vi "Program Synth.vi"(8 "error in (no error)":errorcluster, 11 "NHMFL Synthesizer in":refnum<class "NHMFL Synthesizer.lvclass">) -> (0 "error out":errorcluster, 3 "NHMFL Synthesizer out":refnum<class "NHMFL Synthesizer.lvclass">)   [LabVIEW 2015, in "NHMFL Synthesizer.lvclass"]
uses:
  NHMFL Synthesizer.lvclass
  NHMFL Synthesizer.lvclass/NHMFL Synthesizer.ctl
  Read NHMFL Synthesizer Configuration.vi
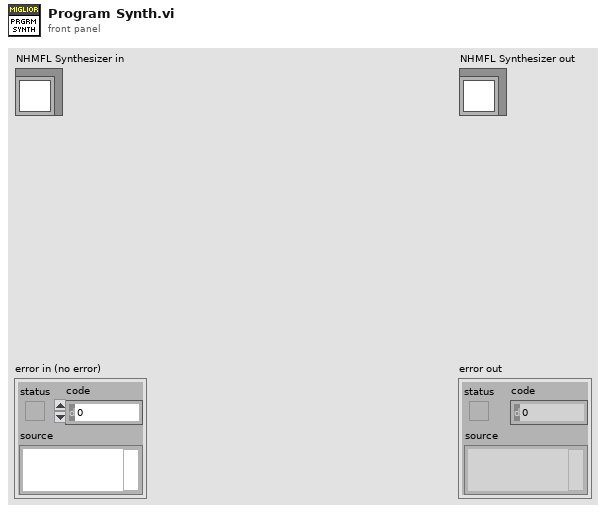
[diagram p1: front panel]
types:
  T1 = typedef "NHMFL Synthesizer Configuration.ctl" = cluster{"DAQmx Device":tag, "Variable amplitude frequency":dbl, "Fixed amplitude frequency":dbl, "Amplitude":dbl, "Clock multiplier":i32, "Cannel names (variable F)":string[], "Cannel names (fixed F)":string[], "Group":string}
  T2 = typedef "Actual settings.ctl" = cluster{"Clock/F1":ext, "Clock/F2":ext, "F1":ext, "F2":ext, "Clock":ext}
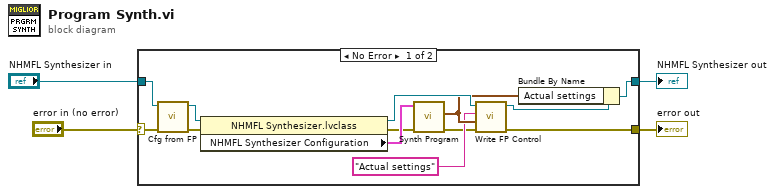
[diagram p0: block diagram]
diagram:
  n1 = case shown="No Error" "error in (no error)" {
    selector: "error in (no error)" -> [w9 w19]
    tunnel: [w10 w19] -> w3
    tunnel: [w15 w18] -> w1
    tunnel: "NHMFL Synthesizer in" -> [w6 w18]
    frame No Error {
      n2 = call-dynamic "Cfg from FP.vi"("error in (no error)"=w9, "Measure Object in"=w6) -> ("error out"=w8:errorcluster, "Measure Object out"=w17:refnum<class "NHMFL Synthesizer.lvclass">)  [unwired: 8 in]
      n3 = property class="NHMFL Synthesizer.lvclass"(reference=w17, error in=w8) -> (reference out=w13:refnum<class "NHMFL Synthesizer.lvclass">, error out=w14:errorcluster, "NHMFL Synthesizer Configuration"=w16:T1)
      n4 = call "Synth Program.vi"("Error In"=w14, "User configuration"=w16) -> ("Error Out"=w7:errorcluster, "Actual ratios"=w12:T2)  [unwired: 7 in, 1 out]
      n5 = call-dynamic "Write FP Control.vi"("error in (no error)"=w7, "Control Value"=w12, "Control Name"="Actual settings", "Measure Object in"=w13) -> ("error out"=w10:errorcluster, "Measure Object out"=w5:refnum<class "NHMFL Synthesizer.lvclass">)  [unwired: 6 in]
      n6 = Bundle By Name(cluster=w5, "Actual settings"=w12) -> (w15:refnum<class "NHMFL Synthesizer.lvclass">)
    }
    frame Error {
    }
  }
  "error out" <- w3
  "NHMFL Synthesizer out" <- w1
